vi "Calcs.vi"(8 "h":dbl format="%#_13g", 9 "T":dbl format="%#_13g", 10 "P":dbl format="%#_13g", 11 "Calcs":T1) -> (1 "Vcorr":dbl, 2 "Vmpt":dbl, 3 "Kpt":dbl)   [LabVIEW 2023, in "GUI.lvlib"]
uses:
  GUI.lvlib
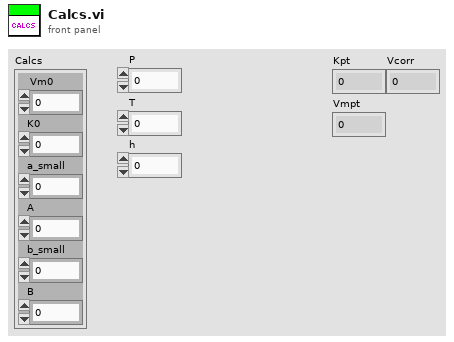
[diagram p1: front panel]
types:
  T1 = cluster{"Vm0":dbl, "K0":dbl, "a_small":dbl, "A":dbl, "b_small":dbl, "B":dbl}
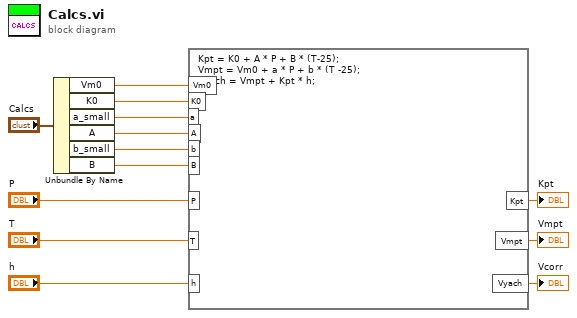
[diagram p0: block diagram]
diagram:
  n1 = Unbundle By Name("Calcs") -> ("Vm0"=w11:dbl, "K0"=w10:dbl, "a_small"=w9:dbl, "A"=w8:dbl, "b_small"=w7:dbl, "B"=w12:dbl)
  n2 = formula code="Kpt = K0 + A * P + B * (T-25);\nVmpt = Vm0 + a * P + b * (T -25);\nVyach = Vmpt + Kpt * h;"("Vm0"=w11, "K0"=w10, "a"=w9, "A"=w8, "b"=w7, "B"=w12, "P"="P", "T"="T", "h"="h") -> ("Kpt"=→"Kpt":dbl, "Vmpt"=→"Vmpt":dbl, "Vyach"=→"Vcorr":dbl)
